vi "Vision-Ball.vi"(10 "Minimum Confidence":dbl=0.15) -> (0 "Confidence":dbl, 1 "z Coordinate of Ball":dbl, 2 "y Coordinate of Ball":dbl, 3 "x Coordinate of Ball":dbl, 5 "ball detected":bool)   [LabVIEW 2015]
uses:
  <vilib>/Analysis/Matrix/Datatypes/RealMatrix.ctl
  Team900-VIs/labview-zmq/socket_type.ctl
  Team900-VIs/labview-zmq/socket_options.ctl
  <vilib>/Analysis/Matrix/Numeric/Conversions/Array To Matrix - RA2.vi
  Team900-VIs/labview-zmq/zmq_socket.lvclass
  Team900-VIs/labview-zmq/zeromq.lvlib
  Team900-VIs/labview-zmq/zmq_context.lvclass
  <vilib>/Analysis/Matrix/NI_Matrix.lvlib
panel:
  in  "Reset":bool
  out "Real Matrix":T1
  in  "Max height":dbl
  out "data":string
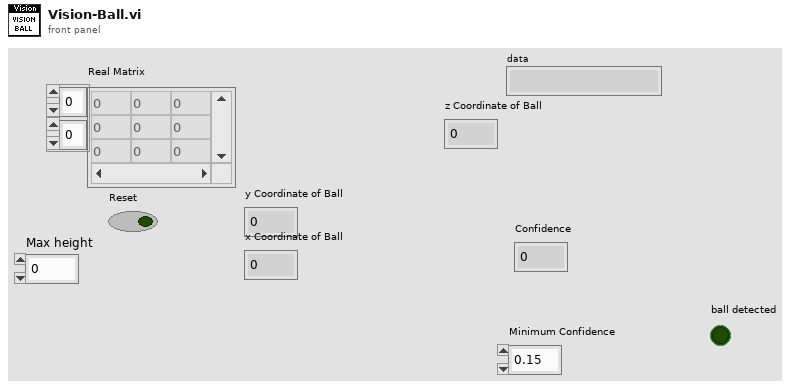
[diagram p1: front panel]
types:
  T1 = typedef "NI_Matrix.lvlib/RealMatrix.ctl" = dbl[][]
  T2 = typedef "zeromq.lvlib/socket_options.ctl" = enum8{"NONE", "ZMQ_HWM", "<2>", "ZMQ_SWAP", "ZMQ_AFFINITY", "ZMQ_IDENTITY", "ZMQ_SUBSCRIBE", "ZMQ_UNSUBSCRIBE", "ZMQ_RATE", "ZMQ_RECOVERY_IVL", "ZMQ_MCAST_LOOP", "ZMQ_SNDBUF", "ZMQ_RCVBUF", "ZMQ_RCVMORE", "ZMQ_FD", "ZMQ_EVENTS", "ZMQ_TYPE", "ZMQ_LINGER", "ZMQ_RECONNECT_IVL", "ZMQ_BACKLOG", "ZMQ_RECOVERY_IVL_MSEC", "ZMQ_RECONNECT_IVL_MAX", "ZMQ_MAXMSGSIZE", "ZMQ_SNDHWM", "ZMQ_RCVHWM", "ZMQ_MULTICAST_HOPS", "<26>", "ZMQ_RCVTIMEO", "ZMQ_SNDTIMEO", "<29>", "<30>", "ZMQ_IPV4ONLY", "ZMQ_LAST_ENDPOINT", "ZMQ_ROUTER_MANDATORY", "ZMQ_TCP_KEEPALIVE", "ZMQ_TCP_KEEPALIVE_CNT", "ZMQ_TCP_KEEPALIVE_IDLE", "ZMQ_TCP_KEEPALIVE_INTVL", "ZMQ_TCP_ACCEPT_FILTER", "ZMQ_DELAY_ATTACH_ON_CONNECT", "ZMQ_XPUB_VERBOSE"}
  T3 = typedef "zeromq.lvlib/socket_type.ctl" = enum8{"ZMQ_PAIR", "ZMQ_PUB", "ZMQ_SUB", "ZMQ_REQ", "ZMQ_REP", "ZMQ_DEALER", "ZMQ_ROUTER", "ZMQ_PULL", "ZMQ_PUSH", "ZMQ_XPUB", "ZMQ_XSUB"}
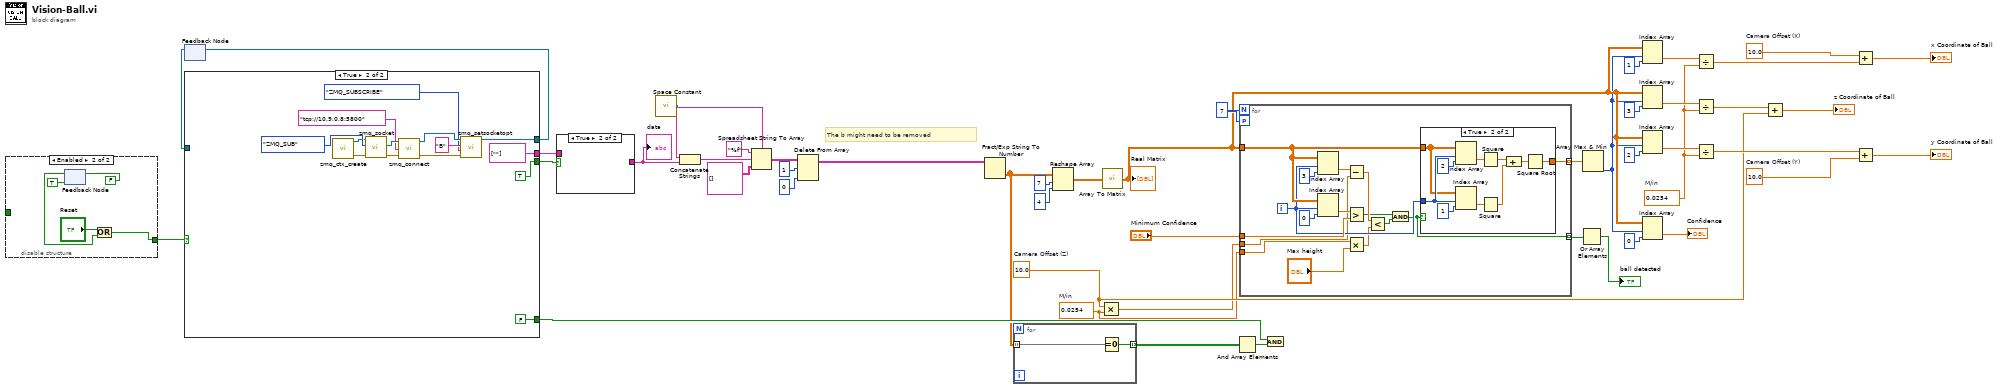
[diagram p0: block diagram]
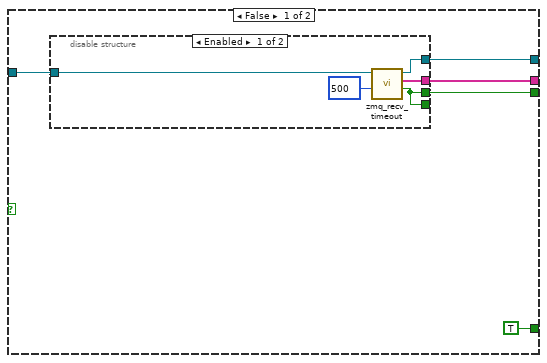
[diagram p2: hidden frame]
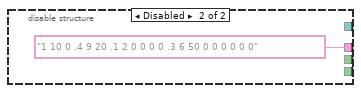
[diagram p3: hidden frame]
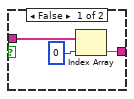
[diagram p4: hidden frame]
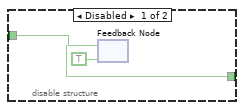
[diagram p5: hidden frame]
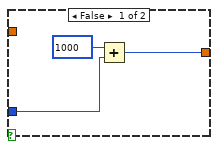
[diagram p6: hidden frame]
diagram:
  w18 = 0.0254  # M/in
  w21 = 0.0254  # M/in
  w17 = 10.0  # Camera Offset (Y)
  w16 = 10.0  # Camera Offset (X)
  w20 = 10.0  # Camera Offset (Z)
  w45 = 7
  # "The b might need to be removed"
  n1 = disable-structure shown="Enabled" {
    disable-tunnel: _ -> [w51 _]
    disable-tunnel: [w49 w54] -> w14
    frame Disabled {
      n2 = feedback #1(TRUE) -> (w49:bool)
      n3 = feedback-in #1(w51) -> ()
    }
    frame Enabled {
      n4 = feedback-in #2(FALSE) -> ()
      n5 = feedback #2(TRUE) -> (w53:bool)
      n6 = Or(x="Reset", y=w53) -> (x .or. y?=w54:bool)
    }
  }
  n7 = feedback #3() -> (w1:refnum<class "zmq_socket.lvclass">)  [unwired: 1 in]
  n8 = case shown="True" w14 {
    tunnel: [w61 string[] [""] ("parts")] -> w4
    tunnel: [w60 TRUE ("timeout?")] -> w3
    tunnel: w1 -> [w59 _]
    tunnel: [w57 w70] -> w2
    tunnel: [TRUE FALSE] -> w35
    frame False {
      n9 = disable-structure shown="Enabled" {
        disable-tunnel: [w66 "1 10 0 .4 9 20 .1 2 0 0 0 0 .3 6 50 0 0 0 0 0 0"] -> w61
        disable-tunnel: [w64 _] -> w60
        disable-tunnel: [w64 _] -> _
        disable-tunnel: w59 -> [w63 _]
        disable-tunnel: [w62 _] -> w57
        frame Enabled {
          n10 = call "zmq_recv_timeout.vi"("timeout (ms)"=u32 500, "socket in"=w63) -> ("timeout?"=w64:bool, "parts"=w66:string[], "socket out"=w62:refnum<class "zmq_socket.lvclass">)  [unwired: 2 in, 1 out]
        }
        frame Disabled {
        }
      }
    }
    frame True {
      n11 = call "zmq_ctx_create.vi"() -> ("error out"=w77:errorcluster, "context out"=w80:refnum<class "zmq_context.lvclass">)  [unwired: 4 in]
      n12 = call "zmq_socket.vi"("error in"=w77, "socket type"=socket_type."ZMQ_SUB", "context in"=w80) -> ("error out"=w74:errorcluster, "socket out"=w79:refnum<class "zmq_socket.lvclass">)  [unwired: 2 in, 1 out]
      n13 = call "zmq_connect.vi"("error in"=w74, "endpoint"="tcp://10.9.0.8:5800" ("Endpoint"), "socket in"=w79) -> ("error out"=w75:errorcluster, "socket out"=w76:refnum<class "zmq_socket.lvclass">)  [unwired: 1 in]
      n14 = call "zmq_setsocketopt.vi"("error in"=w75, "value"="B", "option"=socket_options."ZMQ_SUBSCRIBE", "socket in"=w76) -> ("socket out"=w70:refnum<class "zmq_socket.lvclass">)  [unwired: 2 in, 1 out]
    }
  }
  n15 = feedback-in #3(w2) -> ()
  n16 = case shown="True" w3 {
    tunnel: w4 -> [w84 _]
    tunnel: [w82 _] -> w5
    frame False {
      n17 = Index Array(array=w84, index=0) -> (element=w82:string)
    }
    frame True {
    }
  }
  "data" <- w5
  n18 = call <vilib>:"Space Constant.vi"() -> ("String"=w6:string)
  n19 = Concatenate Strings(w6, w5) -> (w7:string)
  n20 = Spreadsheet String To Array(delimiter (Tab)=w6, format string="%f", spreadsheet string=w7, array type (2D Dbl)=string[][] [] ("Array")) -> (array=w8:string[][])
  n21 = Delete From Array(array=w8, length=1, index (col)=0 ("disabled index (col)")) -> (array with subset deleted=w9:string[][])  [unwired: 1 in, 1 out]
  n22 = Fract/Exp String To Number(string=w9) -> (number=w15:dbl[][])  [unwired: 4 out]
  n23 = for {
    tunnel: w15 -> [w86] mode=indexing
    tunnel: [w85] -> w37 mode=indexing
    n24 = Equal To 0?(x=w86) -> (x = 0?=w85:bool[])
  }
  n25 = Reshape Array(w15, 7 ("dimension size"), 4 ("dimension size")) -> (w46:dbl[][])
  n26 = Multiply(x=w20, y=w18) -> (x*y=w19:dbl)
  n27 = call-poly <vilib>:"Array To Matrix.vi"("Real 2D Array"=w46) -> ("Real Matrix"=w33:T1)
  "Real Matrix" <- w33
  n28 = And Array Elements(Boolean array=w37) -> (logical AND=w36:bool)
  n29 = for {
    N: w45 -> [_]
    workers-P: w45 -> [_]
    tunnel: w33 -> [w97]
    tunnel: "Minimum Confidence" -> [w101]
    tunnel: [w99] -> w43 mode=indexing
    tunnel: [w89] -> w25 mode=indexing
    tunnel: w19 -> [w93]
    tunnel: w18 -> [w87]
    i -> [w96]
    n30 = Index Array(array=w97, index (row)=w96, index (col)=3) -> (element=w95:dbl)
    n31 = Index Array(array=w97, index (row)=w96, index (col)=0) -> (element=w102:dbl)
    n32 = Subtract(x=w95, y=w93) -> (x-y=w94:dbl)
    n33 = Greater?(x=w102, y=w101) -> (0:w91:bool)
    n34 = Multiply(x=w87, y="Max height") -> (x*y=w88:dbl)
    n35 = Less?(x=w94, y=w88) -> (x < y?=w90:bool)
    n36 = And(x=w91, y=w90) -> (x .and. y?=w89:bool)
    n37 = case shown="True" w89 {
      tunnel: w96 -> [w103 w113]
      tunnel: w97 -> [_ w112]
      tunnel: [w104 w106] -> w99
      frame False {
        n38 = Add(x=1000, y=w103) -> (x+y=w104:i32)
      }
      frame True {
        n39 = Index Array(array=w112, index (row)=w113, index (col)=2) -> (element=w111:dbl)
        n40 = Index Array(array=w112, index (row)=w113, index (col)=1) -> (element=w110:dbl)
        n41 = Square(x=w111) -> (x^2=w109:dbl)
        n42 = Square(x=w110) -> (x^2=w108:dbl)
        n43 = Compound Arithmetic op=ADD(w109, w108) -> (w107:dbl)
        n44 = Square Root(x=w107) -> (sqrt(x)=w106:dbl)
      }
    }
  }
  n45 = And(x=w35, y=w36) -> ()  [unwired: 1 out]
  n46 = Or Array Elements(Boolean array=w25) -> (logical OR=→"ball detected":bool)
  n47 = Array Max & Min(array=w43) -> (min index (indices)=w32:i32)  [unwired: 3 out]
  n48 = Index Array(array=w33, index (row)=w32, index (col)=1) -> (element=w31:dbl)
  n49 = Index Array(array=w33, index (row)=w32, index (col)=3) -> (element=w29:dbl)
  n50 = Index Array(array=w33, index (row)=w32, index (col)=2) -> (element=w30:dbl)
  n51 = Index Array(array=w33, index (row)=w32, index (col)=0) -> (element=→"Confidence":dbl)
  n52 = Divide(x=w31, y=w21) -> (x/y=w23:dbl)
  n53 = Divide(x=w29, y=w21) -> (x/y=w22:dbl)
  n54 = Divide(x=w30, y=w21) -> (x/y=w24:dbl)
  n55 = Add(x=w22, y=w20) -> (x+y=→"z Coordinate of Ball":dbl)
  n56 = Add(x=w16, y=w23) -> (x+y=→"x Coordinate of Ball":dbl)
  n57 = Add(x=w24, y=w17) -> (x+y=→"y Coordinate of Ball":dbl)
